vi "1_06.vi"() -> ()   [LabVIEW 2018]
panel:
  in  "Funcion":T1(ring)
  in  "stop":bool
  out "Waveform Chart":dbl[](graph)
  in  "Amplitud":dbl=5.0
  in  "Frecuencia":dbl=1000.0
  in  "Muestras por segundo":dbl=2.0
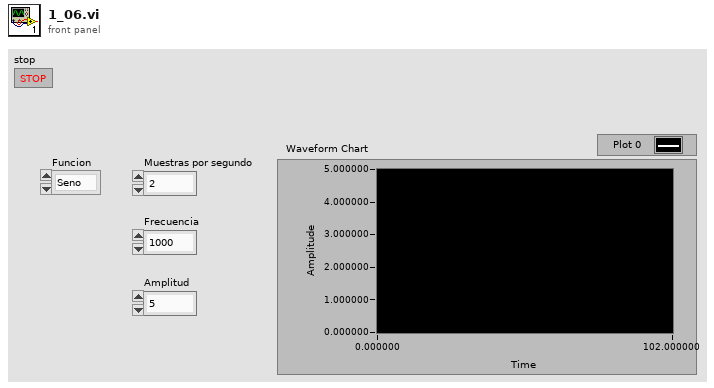
[diagram p1: front panel]
types:
  T1 = enum16{"Seno", "Rampa", "Triangular", "Cuadrada"}
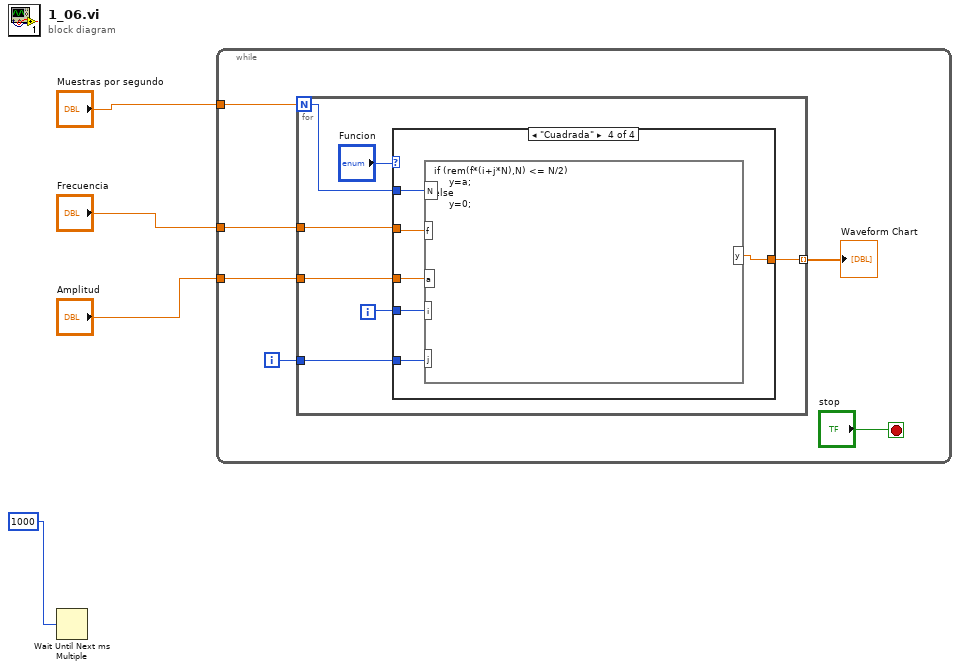
[diagram p0: block diagram]
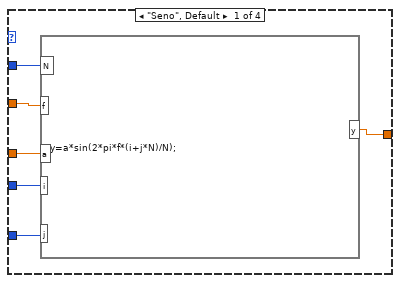
[diagram p2: hidden frame]
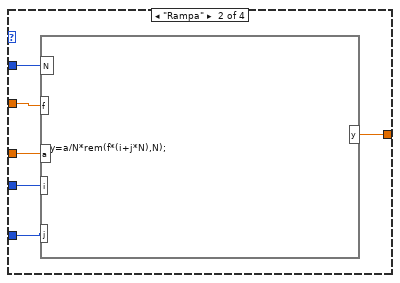
[diagram p3: hidden frame]
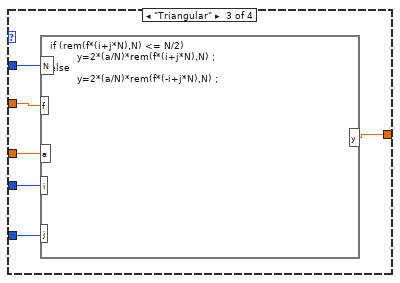
[diagram p4: hidden frame]
diagram:
  n1 = Wait Until Next ms Multiple(millisecond multiple=1000) -> ()  [unwired: 1 out]
  n2 = while {
    tunnel: "Muestras por segundo" -> [w8]
    tunnel: "Frecuencia" -> [w7]
    tunnel: "Amplitud" -> [w6]
    i -> [w9]
    stop <- "stop" stop-if-true
    n3 = for {
      N: w8 -> [w15]
      tunnel: w9 -> [w14]
      tunnel: w7 -> [w12]
      tunnel: w6 -> [w13]
      tunnel: [w11] -> w5 mode=indexing
      i -> [w16]
      n4 = case shown="\"Cuadrada\"" "Funcion" {
        tunnel: w16 -> [w22 w29 w32 w38]
        tunnel: w15 -> [w19 w28 w35 w39]
        tunnel: w14 -> [w23 w27 w31 w37]
        tunnel: w12 -> [w20 w26 w34 w40]
        tunnel: w13 -> [w21 w25 w33 w41]
        tunnel: [w18 w24 w30 w36] -> w11
        frame "Seno", Default {
          n5 = formula code="y=a*sin(2*pi*f*(i+j*N)/N);"("f"=w20, "i"=w22, "j"=w23, "N"=w19, "a"=w21) -> ("y"=w18:dbl)
        }
        frame "Rampa" {
          n6 = formula code="y=a/N*rem(f*(i+j*N),N);"("f"=w26, "i"=w29, "j"=w27, "N"=w28, "a"=w25) -> ("y"=w24:dbl)
        }
        frame "Triangular" {
          n7 = formula code="if (rem(f*(i+j*N),N) <= N/2)\n         y=2*(a/N)*rem(f*(i+j*N),N) ;\nelse\n         y=2*(a/N)*rem(f*(-i+j*N),N) ;"("f"=w34, "i"=w32, "j"=w31, "N"=w35, "a"=w33) -> ("y"=w30:dbl)
        }
        frame "Cuadrada" {
          n8 = formula code="if (rem(f*(i+j*N),N) <= N/2)\n     y=a;\nelse\n     y=0;"("f"=w40, "i"=w38, "j"=w37, "N"=w39, "a"=w41) -> ("y"=w36:dbl)
        }
      }
    }
    "Waveform Chart" <- w5
  }
